vi "thermometer1_api_change_rate.vi"(8 "Sample rate (1-100 Hz)":dbl(knob)=20.0 min=1.0 max=100.0 scale=1.0..100.0, 10 "target (\"thermometer1\")":string="thermometer1", 11 "sender":string) -> ()   [LabVIEW 2019]
doc: "Change the sample rate (Hz) of the <b>target</b> thermometer. Technically, this VI lets you control the sampling frequency but converts it into sampling period (T=1/f, seconds) and sends that value to the target thermometer."
uses:
  common/common data types/common_event_data.ctl
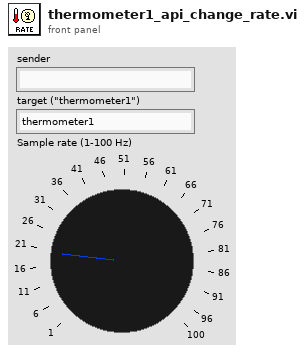
[diagram p1: front panel]
types:
  T1 = typedef "common_event_data.ctl" = cluster{"sender":string, "target":string, "msg":string, "data":variant}
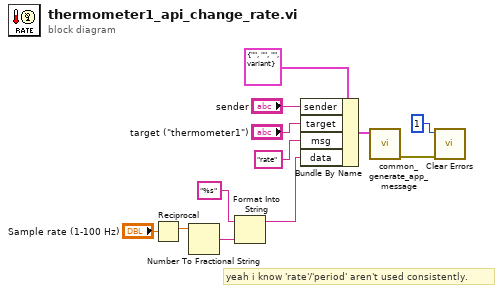
[diagram p0: block diagram]
diagram:
  # "yeah i know 'rate'/'period' aren't used consistently."
  n1 = Reciprocal(x="Sample rate (1-100 Hz)") -> (1/x=w2:dbl)
  n2 = Number To Fractional String(number=w2) -> (F-format string=w1:string)  [unwired: 3 in]
  n3 = Format Into String(format string="%s", w1) -> (resulting string=w7:string)  [unwired: 2 in, 1 out]
  n4 = Bundle By Name(cluster=T1 {"sender"="", "target"="", "msg"="", "data"=variant} ("event data"), "sender"="sender", "target"="target (\"thermometer1\")", "msg"="rate", "data"=w7) -> (w6:T1)
  n5 = call "common_generate_app_message.vi"("event data"=w6) -> ("error out"=w5:errorcluster)  [unwired: 10 in]
  n6 = call <vilib>:"Clear Errors.vi"("error in (no error)"=w5, "specific error code to clear (0: all)"=1) -> ()  [unwired: 4 in, 2 out]
